vi "static.vi"(8 "error in (no error)":errorcluster, 11 "IParent in":refnum<class "IParent.lvclass">) -> (0 "error out":errorcluster, 2 "result":string="IParent's static method is called!", 3 "IParent out":refnum<class "IParent.lvclass">)   [LabVIEW 2024, in "IParent.lvclass"]
uses:
  IParent.lvclass
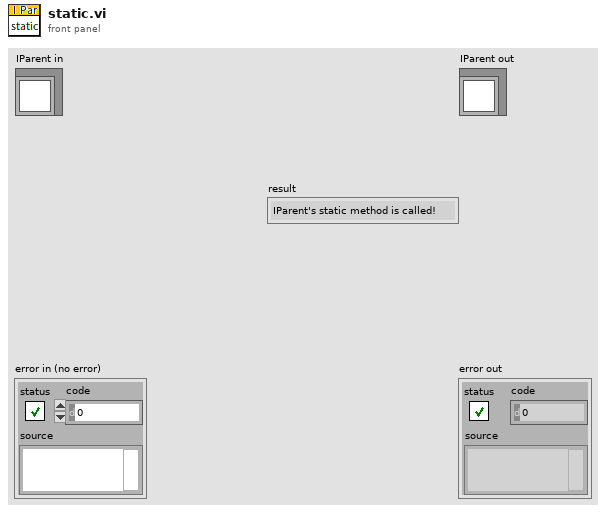
[diagram p1: front panel]
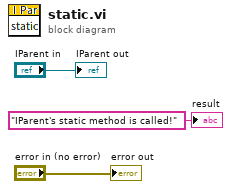
[diagram p0: block diagram]
diagram:
  "error out" <- "error in (no error)"
  "IParent out" <- "IParent in"
  "result" <- "IParent's static method is called!"
